vi "Decimate wfms.vi"(0 "reference in":refnum<class "Fcurve.lvclass">, 2 "Ch Data":waveform(dbl)[](array[waveform]), 5 "error in (no error)":errorcluster) -> (14 "reference out":refnum<class "Fcurve.lvclass">, 16 "Decimated Ch Data":waveform(dbl)[](array[waveform]), 19 "error out":errorcluster)   [LabVIEW 2019, in "Fcurve.lvclass"]
uses:
  Fcurve.lvclass
  <vilib>/Analysis/2dsp.llb/Decimate (single shot, DBL).vi
  <vilib>/Analysis/NI_AALPro.lvlib
panel:
  in  "decimating factor":i32=1
  in  "averaging":bool=TRUE
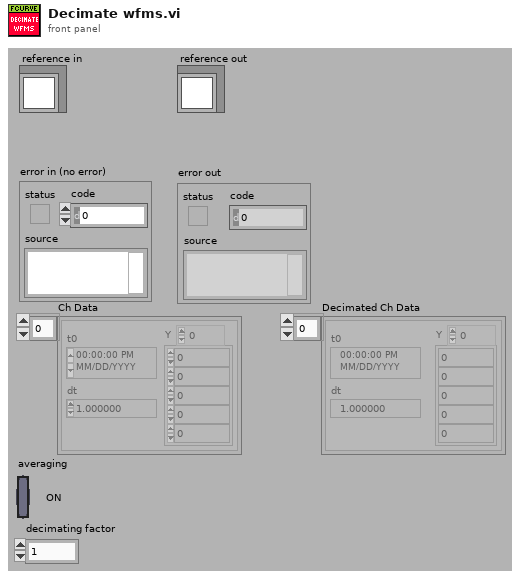
[diagram p1: front panel]
types:
  T1 = typedef "Fcurve.lvclass/ObjectAttributes.ctl" = cluster{"MyAttribute":dbl, "Fcurve Metadata":T2, "Contact Spread of dev":dbl, "Tau Delay (ms)":dbl, "Points of contact":dbl, "Def_wfm":cluster{"Max":dbl, "Min":dbl}, "Zpos_wfm":cluster{"Max":dbl, "Min":dbl}, "Contact stat?":bool, "Real AI dt (s)":dbl, "Decimation":cluster{"App":cluster{"Dec":i32, "apply":bool}, "Con":cluster{"Dec":i32, "apply":bool}, "Ret":cluster{"Dec":i32, "apply":bool}}, "Segment def[0]":dbl, "Segment Zpos[0]":dbl, "Raw Datum":waveform(dbl)[], "Group metadata":T3, "M_data obj":refnum<class "metadata.lvclass">, "Channel name(s)":string[], "Segment fcurve data":cluster{"X":dbl[], "Y":dbl[]}[], "Segment duration":cluster{"Start":i32, "Duration":i32}[], "Segment info":T4[], "Segment durations (S)":dbl[], "Segments Maxmin":T6[]}
  T2 = typedef "Fcurve.lvclass/Metadata.ctl" = cluster{"dt (us)":dbl, "Dec Factor":dbl, "Z piezo Sensitivity (nm/V)":dbl, "K (N/m)":dbl, "Sp (V)":dbl, "Contact (ms)":dbl, "Zpos contact":dbl, "Vel_app (nm/s)":dbl, "Vel_ret (nm/s)":dbl, "deltaV (nm)":dbl, "Def_V0 (v)":dbl, "Piezo gain":dbl, "invOLS (nm/V)":dbl}
  T3 = typedef "TDMS_DataHandler.lvclass/Fcurve Meta data.ctl" = cluster{"property names":string[], "property values":variant[]}
  T4 = typedef "Fcurve.lvclass/Fcurve segments --cluster.ctl" = cluster{"type":T5, "nb points":i32, "dec factor":u32, "sampling rate (S/s)":u32}
  T5 = typedef "metadata.lvclass/Segment type--combobox.ctl" = string
  T6 = typedef "Fcurve.lvclass/Segment MaxMin --cluster.ctl" = cluster{"Def":cluster{"max value":dbl, "min value":dbl}, "Zpos":cluster{"max value":dbl, "min value":dbl}}
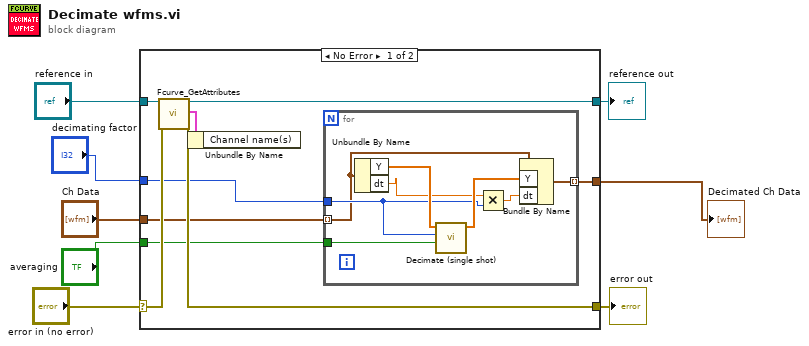
[diagram p0: block diagram]
diagram:
  n1 = case shown="No Error" "error in (no error)" {
    selector: "error in (no error)" -> [w17 w27]
    tunnel: [w16 w27] -> w7
    tunnel: [w15 w26] -> w5
    tunnel: "reference in" -> [w13 w26]
    tunnel: "Ch Data" -> [w12 _]
    tunnel: "averaging" -> [w11 _]
    tunnel: "decimating factor" -> [w10 _]
    tunnel: [w9 _] -> w1
    frame No Error {
      n2 = call "Fcurve_GetAttributes.vi"("reference in"=w13, "error in (no error)"=w17) -> ("reference out"=w15:refnum<class "Fcurve.lvclass">, "attributes"=w14:T1, "error out"=w16:errorcluster)  [unwired: 14 in, 1 out]
      n3 = Unbundle By Name(w14) -> ()  [unwired: 1 out]
      n4 = for {
        tunnel: w12 -> [w18] mode=indexing
        tunnel: w11 -> [w23]
        tunnel: w10 -> [w21]
        tunnel: [w19] -> w9 mode=indexing
        n5 = Unbundle By Name(w18) -> ("Y"=w25:dbl[], "dt"=w22:dbl)
        n6 = call-poly <vilib>:"Decimate (single shot).vi"("averaging"=w23, "decimating factor"=w21, "X"=w25) -> ("Decimated Array"=w24:dbl[])  [unwired: 7 in, 1 out]
        n7 = Multiply(x=w22, y=w21) -> (x*y=w20:dbl)
        n8 = Bundle By Name(cluster=w18, "Y"=w24, "dt"=w20) -> (w19:waveform(dbl))
      }
    }
    frame Error {
    }
  }
  "error out" <- w7
  "reference out" <- w5
  "Decimated Ch Data" <- w1
